vi "INI Get key names.vi"(7 "section":string, 8 "error in":errorcluster) -> (0 "error out":errorcluster, 1 "Found section?":bool, 2 "key names":string[](array[string]), 3 "section names":string[](array[string]))   [LabVIEW 2013]
doc: "This .vi reads the keys from the given section of an .ini file."
uses:
  <vilib>/Utility/config.llb/NI_LVConfig.lvlib
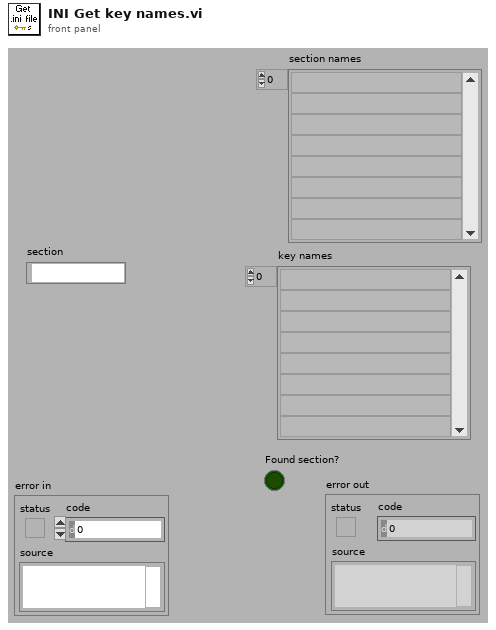
[diagram p1: front panel]
types:
  T1 = typedef "Semaphore RefNum" = refnum<k1>
  T2 = typedef "NI_LVConfig.lvlib/Config Data RefNum.ctl" = refnum<k1>
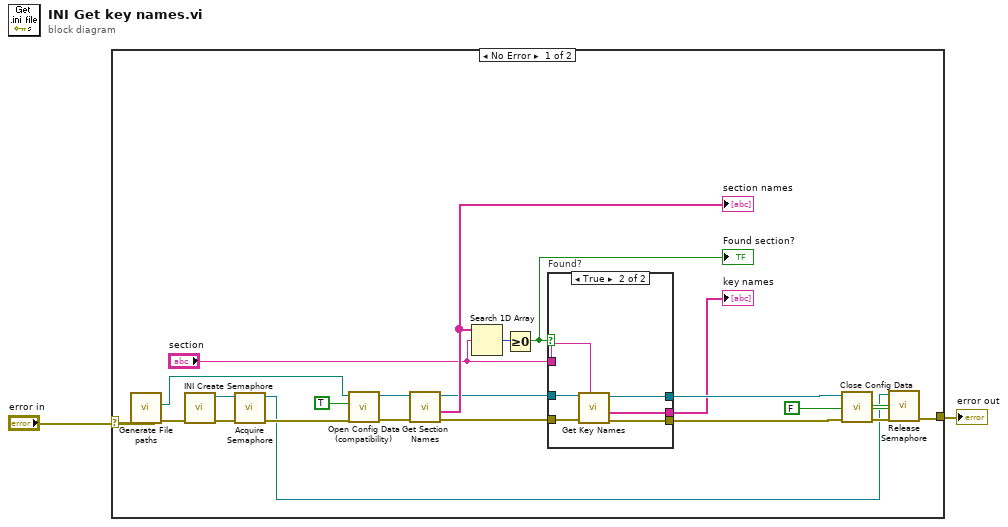
[diagram p0: block diagram]
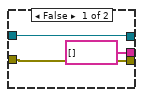
[diagram p2: hidden frame]
diagram:
  n1 = case shown="No Error" "error in" {
    selector: "error in" -> [_ w33]
    tunnel: [w16 w33] -> w1
    frame No Error {
      n2 = call "Generate File paths.vi"() -> ("error out"=w4:errorcluster, ".ini path"=w3:path)  [unwired: 1 in, 9 out]
      n3 = call "INI Create Semaphore.vi"("error in"=w4) -> ("error out"=w21:errorcluster, "semaphore"=w20:T1)  [unwired: 1 in, 4 out]
      n4 = call <vilib>:"Acquire Semaphore.vi"("error in (no error)"=w21, "semaphore"=w20) -> ("error out"=w19:errorcluster, "semaphore out"=w17:T1)  [unwired: 1 in, 3 out]
      n5 = call <vilib>:"Open Config Data (compatibility).vi"("error in (no error)"=w19, "create file if necessary (T)"=TRUE ("create file if necessary? (T)"), "configuration file path"=w3) -> ("error out"=w15:errorcluster, "refnum"=w14:T2)  [unwired: 6 in, 1 out]
      n6 = call <vilib>:"Get Section Names.vi"("error in (no error)"=w15, "refnum"=w14) -> ("error out"=w11:errorcluster, "section names"=w13:string[], "refnum out"=w12:T2)  [unwired: 7 out]
      "section names" <- w13
      n7 = Search 1D Array(1D array=w13, element="section") -> (index of element=w9:i32)  [unwired: 1 out]
      n8 = Greater Or Equal To 0?(x=w9) -> (x >= 0?=w5:bool)
      "Found section?" <- w5
      n9 = case "Found?" shown="True" w5 {
        tunnel: w12 -> [w26 w32]
        tunnel: w11 -> [w25 w31]
        tunnel: "section" -> [_ w30]
        tunnel: [w25 w29] -> w8
        tunnel: [w26 w28] -> w7
        tunnel: [string[] [] ("key names") w27] -> w6
        frame False {
        }
        frame True {
          n10 = call <vilib>:"Get Key Names.vi"("section"=w30, "error in (no error)"=w31, "refnum"=w32) -> ("error out"=w29:errorcluster, "key names"=w27:string[], "refnum out"=w28:T2)  [unwired: 6 out]
        }
      }
      "key names" <- w6
      n11 = call <vilib>:"Close Config Data.vi"("error in (no error)"=w8, "write file if changed (T)"=FALSE ("write configuration file? (T)"), "refnum"=w7) -> ("error out"=w18:errorcluster)  [unwired: 8 out]
      n12 = call <vilib>:"Release Semaphore.vi"("error in (no error)"=w18, "semaphore"=w17) -> ("error out"=w16:errorcluster)  [unwired: 5 out]
    }
    frame Error {
    }
  }
  "error out" <- w1
